vi "Write Bool.vi"(8 "error in (no error)":errorcluster, 10 "Bool":bool, 11 "Generic Boolean Message in":refnum<class "Generic Boolean Message.lvclass">) -> (0 "error out":errorcluster, 3 "Generic Boolean Message out":refnum<class "Generic Boolean Message.lvclass">)   [LabVIEW 2016, in "Controller.lvlib" / "Generic Boolean Message.lvclass"]
uses:
  Generic Boolean Message.lvclass
  Generic Boolean Message.lvclass/Generic Boolean Message.ctl
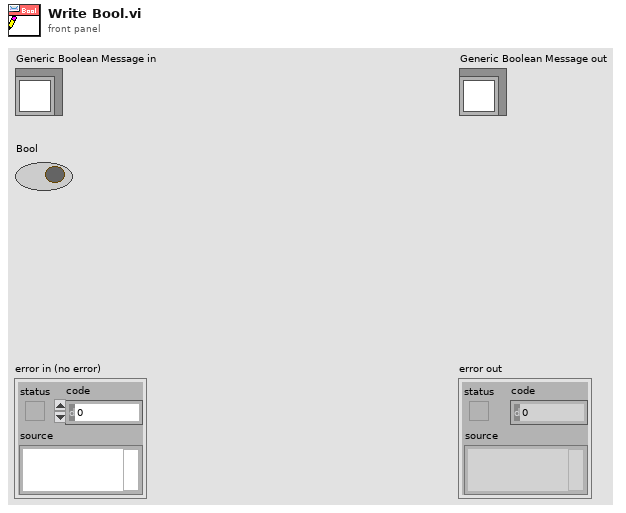
[diagram p1: front panel]
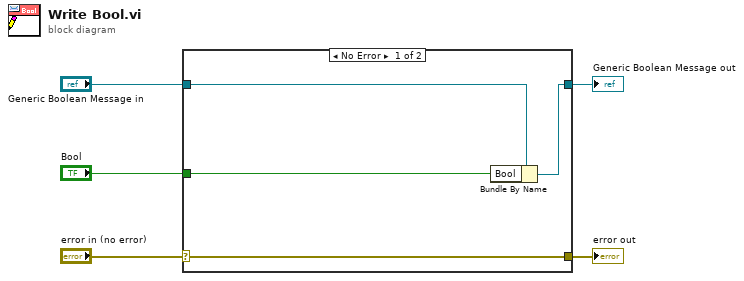
[diagram p0: block diagram]
diagram:
  n1 = case shown="No Error" "error in (no error)" {
    selector: "error in (no error)" -> [w9 w10]
    tunnel: [w9 w10] -> w4
    tunnel: [w7 w11] -> w2
    tunnel: "Generic Boolean Message in" -> [w8 w11]
    tunnel: "Bool" -> [w6 _]
    frame No Error {
      n2 = Bundle By Name(cluster=w8, "Bool"=w6) -> (w7:refnum<class "Generic Boolean Message.lvclass">)
    }
    frame Error {
    }
  }
  "error out" <- w4
  "Generic Boolean Message out" <- w2
